vi "Write Status.vi"(8 "error in (no error)":errorcluster, 10 "Guider Contents":T1, 11 "Guider in":refnum<class "Guider.lvclass">) -> (0 "error out":errorcluster, 3 "Guider out":refnum<class "Guider.lvclass">)   [LabVIEW 2018, in "Guider.lvclass"]
uses:
  Guider.lvclass
  Guider.lvclass/Guider.ctl
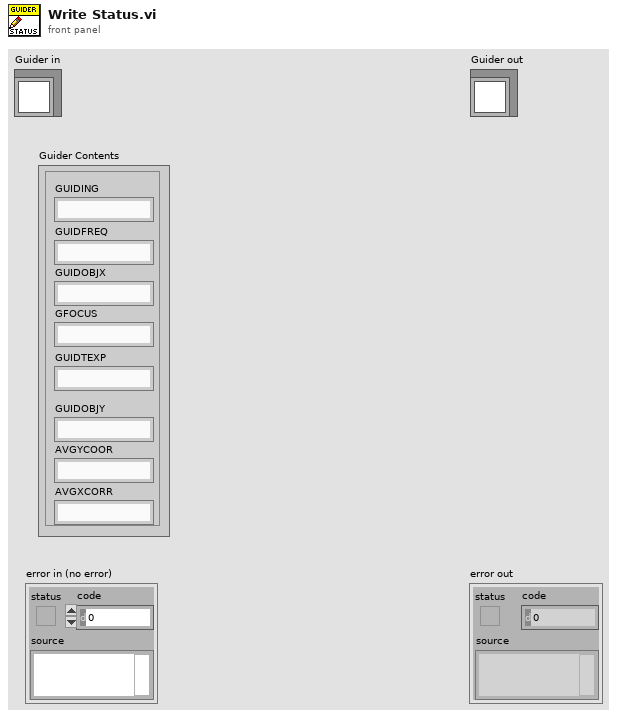
[diagram p1: front panel]
types:
  T1 = cluster{"GUIDING":string, "GUIDTEXP":string, "GUIDFREQ":string, "GUIDOBJX":string, "GUIDOBJY":string, "AVGYCOOR":string, "AVGXCORR":string, "GFOCUS":string}
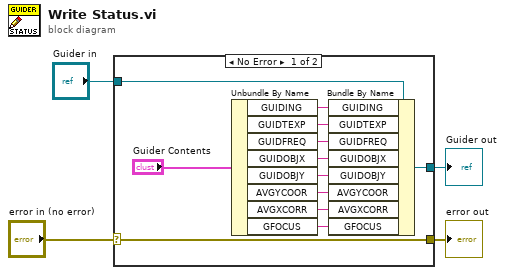
[diagram p0: block diagram]
diagram:
  n1 = case shown="No Error" "error in (no error)" {
    selector: "error in (no error)" -> [w16 w18]
    tunnel: [w16 w18] -> w3
    tunnel: [w13 w17] -> w1
    tunnel: "Guider in" -> [w14 w17]
    frame No Error {
      n2 = Unbundle By Name("Guider Contents") -> ("GUIDING"=w5:string, "GUIDTEXP"=w6:string, "GUIDFREQ"=w7:string, "GUIDOBJX"=w8:string, "GUIDOBJY"=w9:string, "AVGYCOOR"=w10:string, "AVGXCORR"=w11:string, "GFOCUS"=w12:string)
      n3 = Bundle By Name(cluster=w14, "GUIDING"=w5, "GUIDTEXP"=w6, "GUIDFREQ"=w7, "GUIDOBJX"=w8, "GUIDOBJY"=w9, "AVGYCOOR"=w10, "AVGXCORR"=w11, "GFOCUS"=w12) -> (w13:refnum<class "Guider.lvclass">)
    }
    frame Error {
    }
  }
  "error out" <- w3
  "Guider out" <- w1
